vi "Set Fetch Times.vi"(8 "error in (no error)":errorcluster, 10 "Fetch Step In":refnum<k7>, 11 "SPECAN_PVT in":refnum<class "SPECAN_PVT.lvclass">) -> (0 "error out":errorcluster, 2 "Step Out":refnum<k7>, 3 "SPECAN_PVT out":refnum<class "SPECAN_PVT.lvclass">)   [LabVIEW 2018, in "SPECAN_PVT.lvlib" / "SPECAN_PVT.lvclass"]
uses:
  SPECAN_PVT.lvclass
  C:/Sequence Automation/Plugins/Measurement Interface.lvlibp/Measurement Interface.lvclass
  SPECAN_PVT.lvclass/SPECAN_PVT.ctl
  Read Transition Type.vi
  Read Measurement Times.vi
  Plugins/Measurement Interface.lvlibp/Private Methods/Engine Reference/Read Engine Reference.vi
  Plugins/TestStand API Tools (TSAT).lvlibp/Step Actions/TSAT Step Actions.lvlib
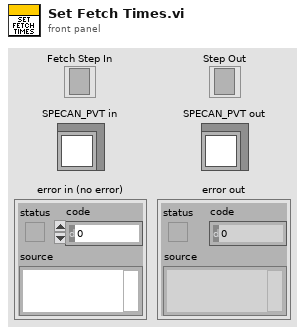
[diagram p1: front panel]
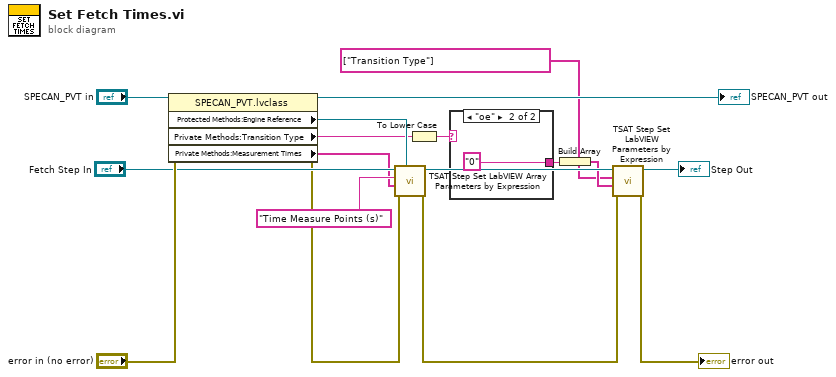
[diagram p0: block diagram]
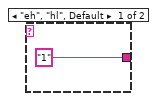
[diagram p2: hidden frame]
diagram:
  n1 = property class="SPECAN_PVT.lvclass"(reference="SPECAN_PVT in", error in="error in (no error)") -> (reference out=→"SPECAN_PVT out":refnum<class "SPECAN_PVT.lvclass">, error out=w12:errorcluster, "Protected Methods:Engine Reference"=w14:refnum<k7>, "Private Methods:Transition Type"=w7:string, "Private Methods:Measurement Times"=w8:string[])
  n2 = call "TSAT Step Set LabVIEW Array Parameters by Expression.vi"("Engine In"=w14, "Error In"=w12, "Value Expressions"=w8, "Parameter to Set"="Time Measure Points (s)", "Step In"="Fetch Step In") -> ("Error Out"=w2:errorcluster, "Step Out"=w10:refnum<k7>)  [unwired: 5 in]
  n3 = To Lower Case(string=w7) -> (all lower case string=w6:string)
  n4 = case shown="\"oe\"" w6 {
    tunnel: ["1" "0"] -> w5
    frame "eh", "hl", Default {
    }
    frame "oe" {
    }
  }
  n5 = Build Array(w5) -> (w4:string[])
  n6 = call "TSAT Step Set LabVIEW Parameters by Expression.vi"("Error In"=w2, "Value Expressions"=w4, "Parameters to Set"=string[] ["Transition Type"], "Step In"=w10) -> ("Error Out"=→"error out":errorcluster, "Step Out"=→"Step Out":refnum<k7>)  [unwired: 6 in]
